vi "ws Data Folder.vi"(3 "Relative Path (\"\" - Folder)":string) -> (1 "Data Folder":path)   [LabVIEW 2011]
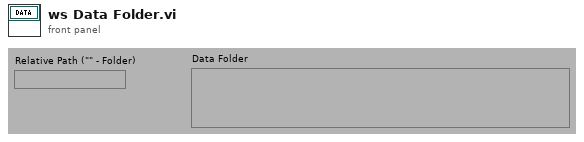
[diagram p1: front panel]
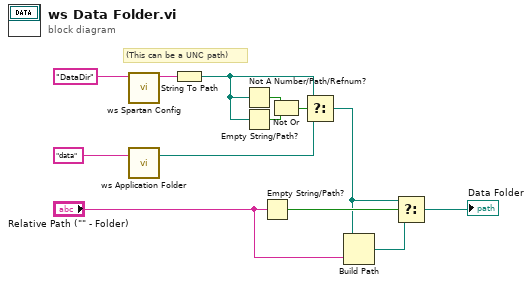
[diagram p0: block diagram]
diagram:
  # "(This can be a UNC path)"
  n1 = call "ws Spartan Config.vi"("config key (\"\")"="DataDir" ("name or relative path")) -> ("config value"=w1:string)  [unwired: 8 in, 2 out]
  n2 = call "ws Application Folder.vi"("Relative Path (\"\" - Folder)"="data" ("name or relative path")) -> ("Application Folder"=w3:path)  [unwired: 2 in]
  n3 = String To Path(string=w1) -> (path=w5:path)
  n4 = Not A Number/Path/Refnum?(number/path/refnum=w5) -> (NaN/Path/Refnum?=w7:bool)
  n5 = Empty String/Path?(string/path=w5) -> (empty?=w8:bool)
  n6 = Empty String/Path?(string/path="Relative Path (\"\" - Folder)") -> (empty?=w12:bool)
  n7 = Not Or(1:w8, 2:w7) -> (0:w6:bool)
  n8 = Select(t=w5, s=w6, f=w3) -> (s? t:f=w9:path)
  n9 = Build Path(base path=w9, name or relative path="Relative Path (\"\" - Folder)") -> (appended path=w10:path)
  n10 = Select(t=w9, s=w12, f=w10) -> (s? t:f=→"Data Folder":path)
